vi "CHROMA Send Receive Multi.vi"(8 "Error In":errorcluster, 10 "Array of Commands":string[](array[string]), 11 "CHROMA VISA In":refnum<visa-resource-name>) -> (0 "Error Out":errorcluster, 2 "Array of Results":string[](array[string]), 3 "CHROMA VISA Out":refnum<visa-resource-name>)   [LabVIEW 2016]
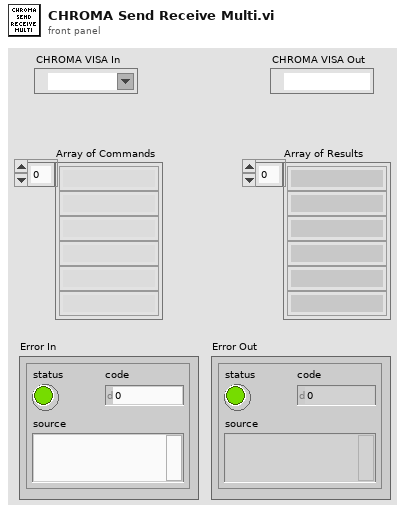
[diagram p1: front panel]
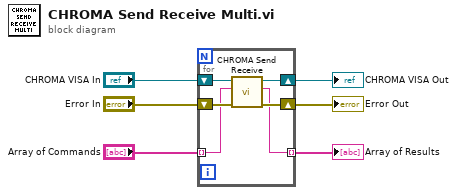
[diagram p0: block diagram]
diagram:
  n1 = for {
    tunnel: "Array of Commands" -> [w9] mode=indexing
    shift-right: [w12] -> w2
    shift-left: "CHROMA VISA In" -> [w10]
    shift-right: [w8] -> w5
    shift-left: "Error In" -> [w11]
    tunnel: [w7] -> w3 mode=indexing
    n2 = call "CHROMA Send Receive.vi"("error in (no error)"=w11, "Send Command"=w9, "CHROMA VISA In"=w10) -> ("error out"=w8:errorcluster, "read buffer"=w7:string, "CHROMA VISA Out"=w12:refnum<visa-resource-name>)  [unwired: 6 in]
  }
  "Error Out" <- w5
  "Array of Results" <- w3
  "CHROMA VISA Out" <- w2
